vi "Equip-Save config.vi"(0 "Slots":T3(array[cluster]) {"Output sources" items=["--unused--", "Right primary", "Right secondary", "Left primary", "Left secondary", "Shocks", "Startle", "Background", "Shaker", "Blue laser"]; "Input sources" items=["--unused--", "Probe Mic Right", "Probe Mic Left", "Cal Mic", "ABR", "CAP Right", "CAP Left", "Startle piezo", "Temperature", "Heart rate", "Accelerometer", "Startle piezo 2"]}, 5 "config name":string, 11 "error in (no error)":errorcluster) -> (15 "error out":errorcluster)   [LabVIEW 2020]
uses:
  Type Defs/Output sources.ctl
  Type Defs/Input sources.ctl
  <vilib>/Utility/config.llb/Write Key (I32).vi
  <vilib>/Utility/config.llb/NI_LVConfig.lvlib
panel:
  in  "Input sources":T1 items=["--unused--", "Probe Mic Right", "Probe Mic Left", "Cal Mic", "ABR", "CAP Right", "CAP Left", "Startle piezo", "Temperature", "Heart rate", "Accelerometer", "Startle piezo 2"]
  in  "Output sources":T2 items=["--unused--", "Right primary", "Right secondary", "Left primary", "Left secondary", "Shocks", "Startle", "Background", "Shaker", "Blue laser"]
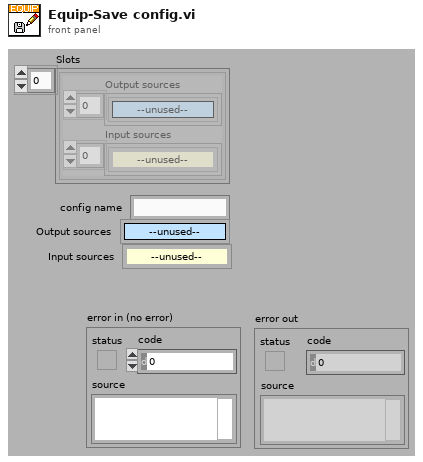
[diagram p1: front panel]
types:
  T1 = typedef "Input sources.ctl" = u16
  T2 = typedef "Output sources.ctl" = u16
  T3 = cluster{"Output sources":T2[], "Input sources":T1[]}[]
  T4 = typedef "NI_LVConfig.lvlib/Config Data RefNum.ctl" = refnum<k1>
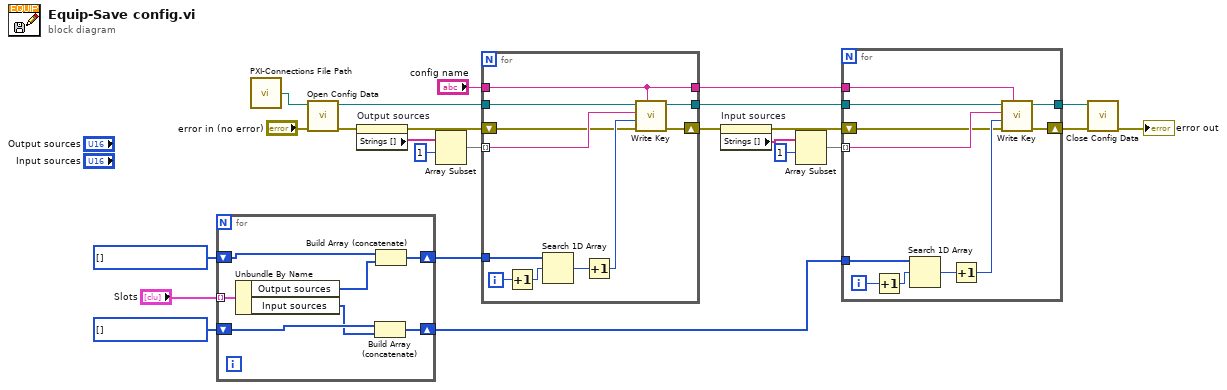
[diagram p0: block diagram]
diagram:
  w22 = T1[] [] items=["--unused--", "Probe Mic Right", "Probe Mic Left", "Cal Mic", "ABR", "CAP Right", "CAP Left", "Startle piezo", "Temperature", "Heart rate"]
  w23 = T2[] [] items=["--unused--", "Right primary", "Right secondary", "Left primary", "Left secondary", "Shocks", "Startle", "Background"]
  n1 = for {
    tunnel: "Slots" -> [w31] mode=indexing
    shift-right: [w29] -> w18
    shift-left: w23 -> [w28]
    shift-right: [w27] -> w8
    shift-left: w22 -> [w26]
    n2 = Unbundle By Name(w31) -> ("Output sources"=w30:T2[], "Input sources"=w25:T1[])
    n3 = Build Array (concatenate)(w26, w25) -> (w27:T1[])
    n4 = Build Array (concatenate)(w28, w30) -> (w29:T2[])
  }
  n5 = call "PXI-Connections File Path.vi"() -> ("Path"=w1:path)  [unwired: 1 in]
  n6 = call <vilib>:"Open Config Data.vi"("error in (no error)"="error in (no error)", "configuration file path"=w1) -> ("error out"=w13:errorcluster, "refnum"=w17:T4)  [unwired: 7 in, 1 out]
  n7 = property on="Output sources" class="Ring (strict)"(error in=w13) -> (error out=w12:errorcluster, "Strings []"=w20:string[])  [unwired: 1 in, 1 out]
  n8 = Array Subset(array=w20, index=1) -> (w21:string[])  [unwired: 1 in]
  n9 = for {
    tunnel: w21 -> [w37] mode=indexing
    tunnel: w18 -> [w42]
    tunnel: w17 -> [w38]
    tunnel: "config name" -> [w32]
    shift-right: [w34] -> w14
    shift-left: w12 -> [w35]
    tunnel: [w33] -> w7
    tunnel: [w32] -> w6
    i -> [w41]
    n10 = Increment(x=w41) -> (x+1=w40:i32)
    n11 = Search 1D Array(1D array=w42, element=w40) -> (index of element=w39:i32)  [unwired: 1 in]
    n12 = Increment(x=w39) -> (x+1=w36:i32)
    n13 = call-poly <vilib>:"Write Key.vi"("section"=w32, "error in (no error)"=w35, "value"=w36, "key"=w37, "refnum"=w38) -> ("error out"=w34:errorcluster, "refnum out"=w33:T4)  [unwired: 4 in, 1 out]
  }
  n14 = property on="Input sources" class="Ring (strict)"(error in=w14) -> (error out=w5:errorcluster, "Strings []"=w10:string[])  [unwired: 1 in, 1 out]
  n15 = Array Subset(array=w10, index=1) -> (w9:string[])  [unwired: 1 in]
  n16 = for {
    tunnel: w9 -> [w47] mode=indexing
    tunnel: w8 -> [w50]
    tunnel: w7 -> [w49]
    tunnel: w6 -> [w48]
    tunnel: [w44] -> w4
    shift-right: [w43] -> w3
    shift-left: w5 -> [w45]
    i -> [w51]
    n17 = Increment(x=w51) -> (x+1=w53:i32)
    n18 = Search 1D Array(1D array=w50, element=w53) -> (index of element=w52:i32)  [unwired: 1 in]
    n19 = Increment(x=w52) -> (x+1=w46:i32)
    n20 = call-poly <vilib>:"Write Key.vi"("section"=w48, "error in (no error)"=w45, "value"=w46, "key"=w47, "refnum"=w49) -> ("error out"=w43:errorcluster, "refnum out"=w44:T4)  [unwired: 4 in, 1 out]
  }
  n21 = call <vilib>:"Close Config Data.vi"("error in (no error)"=w3, "refnum"=w4) -> ("error out"=→"error out":errorcluster)  [unwired: 8 in, 1 out]
